vi "Limit Switches.vi"(11 "State Control":enum16{"Open", "Run", "End"}(ring)) -> (0 "Shooter Top":bool, 1 "Shooter Bottom":bool, 2 "Picker Upper Bottom":bool, 3 "Picker Upper Top":bool)   [LabVIEW 2013]
uses:
  <vilib>/Rock Robotics/SystemInterfaces/DIO/FPGA_DIOChannel.ctl
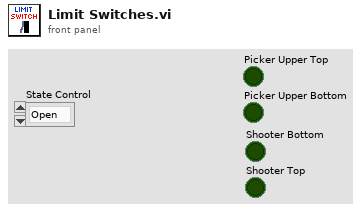
[diagram p1: front panel]
types:
  T1 = typedef "FPGA_DIOChannel.ctl" = enum8{"DIO 1", "DIO 2", "DIO 3", "DIO 4", "DIO 5", "DIO 6", "DIO 7", "DIO 8", "DIO 9", "DIO 10", "DIO 11", "DIO 12", "DIO 13", "DIO 14", "Invalid"}
  T2 = typedef "WPI_DigitalInputDevRef.ctl" = cluster{"DevStatus":errorcluster, "DIO Channel":T1, "Digital Module":T3}
  T3 = typedef "FPGA_TypedefDigitalModule.ctl" = enum16{"Digital Module 1", "Digital Module 2"}
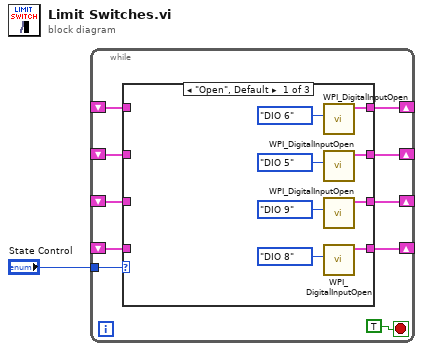
[diagram p0: block diagram]
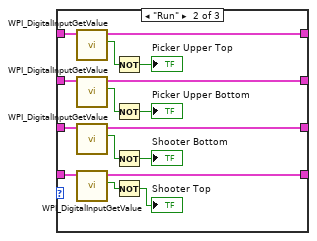
[diagram p2: hidden frame]
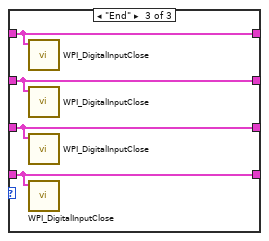
[diagram p3: hidden frame]
diagram:
  n1 = while {
    tunnel: "State Control" -> [w11]
    shift-right: [w9] -> _
    shift-left: _ -> [w7]
    shift-right: [w8] -> _
    shift-left: _ -> [w6]
    shift-right: [w5] -> _
    shift-left: _ -> [w3]
    shift-right: [w4] -> _
    shift-left: _ -> [w2]
    stop <- TRUE stop-if-true
    n2 = case shown="\"Open\", Default" w11 {
      tunnel: [w17 w32 w39] -> w9
      tunnel: [w16 w33 w38] -> w8
      tunnel: w7 -> [_ w35 w39]
      tunnel: w6 -> [_ w34 w38]
      tunnel: [w13 w28 w37] -> w5
      tunnel: [w12 w29 w36] -> w4
      tunnel: w3 -> [_ w31 w37]
      tunnel: w2 -> [_ w30 w36]
      frame "Open", Default {
        n3 = call <vilib>:"WPI_DigitalInputOpen.vi"("DIO Channel"=FPGA_DIOChannel."DIO 6") -> ("DigitalInputDevRef"=w17:T2)  [unwired: 2 in, 8 out]
        n4 = call <vilib>:"WPI_DigitalInputOpen.vi"("DIO Channel"=FPGA_DIOChannel."DIO 5") -> ("DigitalInputDevRef"=w16:T2)  [unwired: 2 in, 8 out]
        n5 = call <vilib>:"WPI_DigitalInputOpen.vi"("DIO Channel"=FPGA_DIOChannel."DIO 9") -> ("DigitalInputDevRef"=w13:T2)  [unwired: 2 in, 8 out]
        n6 = call <vilib>:"WPI_DigitalInputOpen.vi"("DIO Channel"=FPGA_DIOChannel."DIO 8") -> ("DigitalInputDevRef"=w12:T2)  [unwired: 2 in, 8 out]
      }
      frame "Run" {
        n7 = call <vilib>:"WPI_DigitalInputGetValue.vi"("DigitalInputDevRef"=w35) -> ("Value"=w27:bool, "DigitalInputDevRef"=w32:T2)  [unwired: 1 in, 8 out]
        n8 = call <vilib>:"WPI_DigitalInputGetValue.vi"("DigitalInputDevRef"=w34) -> ("Value"=w25:bool, "DigitalInputDevRef"=w33:T2)  [unwired: 1 in, 8 out]
        n9 = call <vilib>:"WPI_DigitalInputGetValue.vi"("DigitalInputDevRef"=w31) -> ("Value"=w23:bool, "DigitalInputDevRef"=w28:T2)  [unwired: 1 in, 8 out]
        n10 = call <vilib>:"WPI_DigitalInputGetValue.vi"("DigitalInputDevRef"=w30) -> ("Value"=w21:bool, "DigitalInputDevRef"=w29:T2)  [unwired: 1 in, 8 out]
        n11 = Not(x=w27) -> (.not. x?=→"Picker Upper Top":bool)
        n12 = Not(x=w25) -> (.not. x?=→"Picker Upper Bottom":bool)
        n13 = Not(x=w23) -> (.not. x?=→"Shooter Bottom":bool)
        n14 = Not(x=w21) -> (.not. x?=→"Shooter Top":bool)
      }
      frame "End" {
        n15 = call <vilib>:"WPI_DigitalInputClose.vi"("DigitalInputDevRef"=w39) -> ()  [unwired: 10 in, 1 out]
        n16 = call <vilib>:"WPI_DigitalInputClose.vi"("DigitalInputDevRef"=w38) -> ()  [unwired: 10 in, 1 out]
        n17 = call <vilib>:"WPI_DigitalInputClose.vi"("DigitalInputDevRef"=w37) -> ()  [unwired: 10 in, 1 out]
        n18 = call <vilib>:"WPI_DigitalInputClose.vi"("DigitalInputDevRef"=w36) -> ()  [unwired: 10 in, 1 out]
      }
    }
  }
